vi "Red_Micro_Parse.vi"(10 "Data":string, 11 "Redundant Micro in":T1) -> (3 "Redundant Micro out":T1)   [LabVIEW 2016]
uses:
  type defs/Redundant.ctl
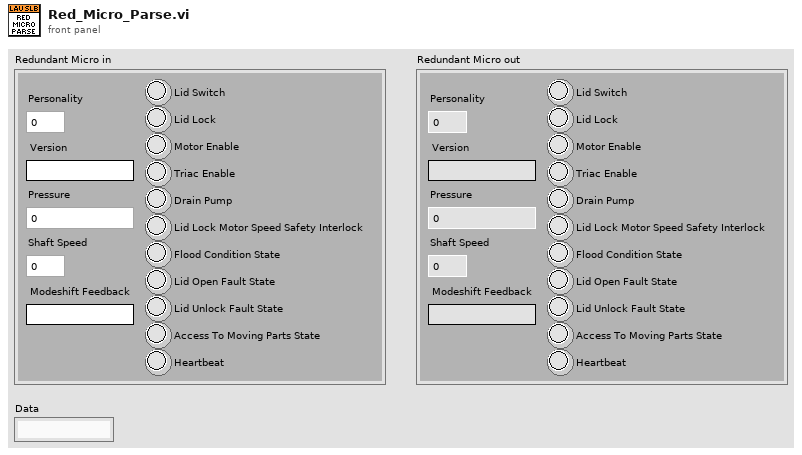
[diagram p1: front panel]
types:
  T1 = typedef "Redundant.ctl" = cluster{"Version":string, "Personality":u8, "Pressure ":dbl, "Shaft Speed":u16, "Modeshift Feedback":string, "Lid Switch":bool, "Lid Lock":bool, "Triac Enable":bool, "Drain Pump":bool, "Lid Lock Motor Speed Safety Interlock":bool, "Flood Condition State":bool, "Lid Open Fault State":bool, "Access To Moving Parts State":bool, "Heartbeat":bool, "Motor Enable":bool, "Lid Unlock Fault State":bool}
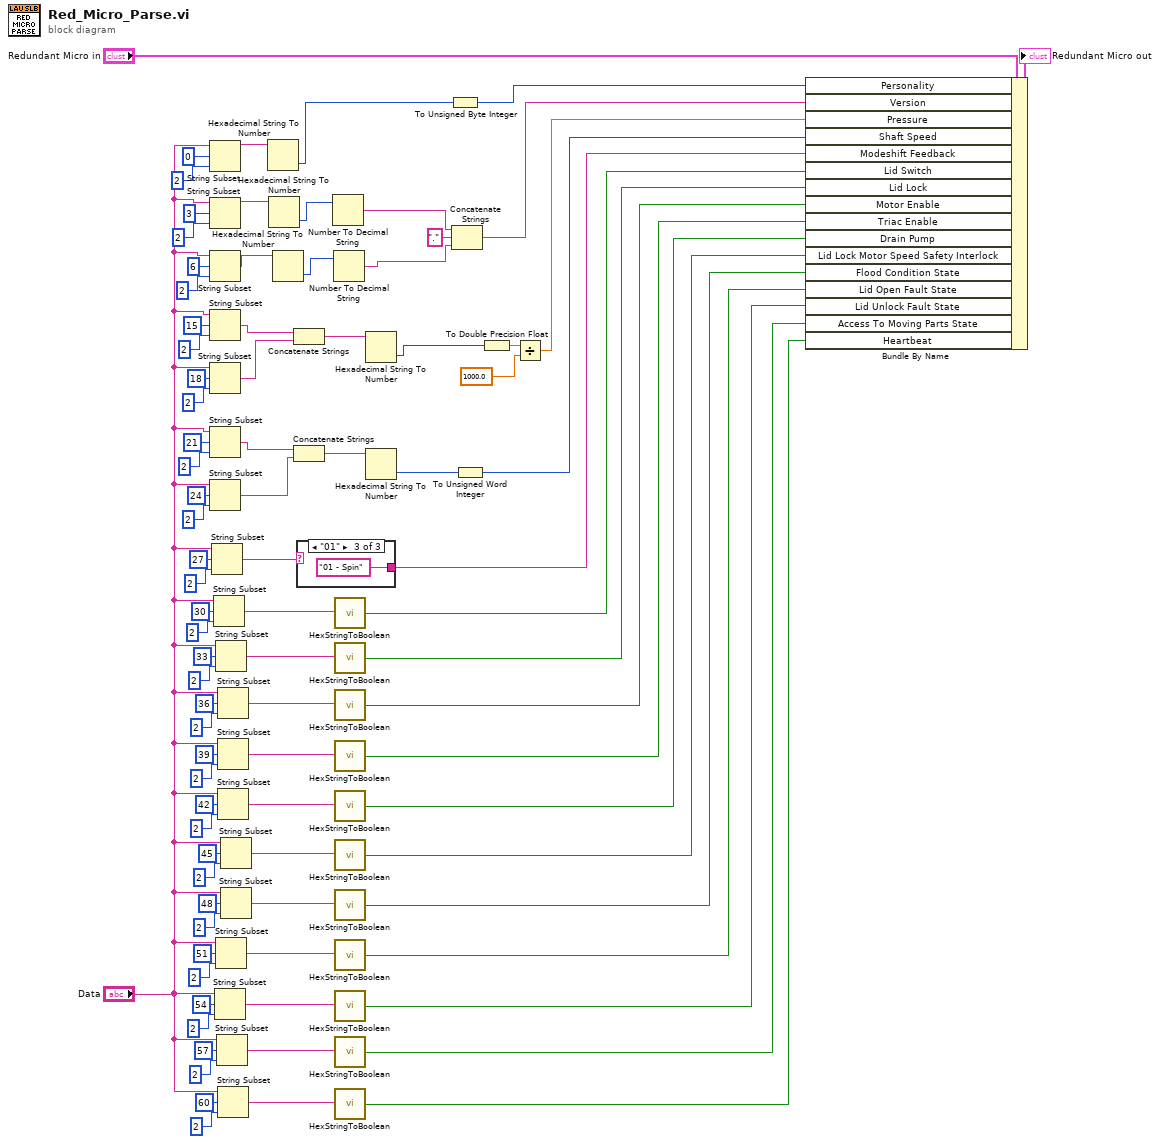
[diagram p0: block diagram]
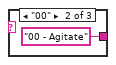
[diagram p3: hidden frame]
diagram:
  n1 = String Subset(string="Data", offset (0)=0, length (rest)=2 ("length (rest)")) -> (substring=w3:string)
  n2 = String Subset(string="Data", offset (0)=3, length (rest)=2 ("length (rest)")) -> (substring=w5:string)
  n3 = String Subset(string="Data", offset (0)=6, length (rest)=2 ("length (rest)")) -> (substring=w11:string)
  n4 = String Subset(string="Data", offset (0)=15, length (rest)=2 ("length (rest)")) -> (substring=w22:string)
  n5 = String Subset(string="Data", offset (0)=18, length (rest)=2 ("length (rest)")) -> (substring=w23:string)
  n6 = String Subset(string="Data", offset (0)=21, length (rest)=2 ("length (rest)")) -> (substring=w31:string)
  n7 = String Subset(string="Data", offset (0)=24, length (rest)=2 ("length (rest)")) -> (substring=w32:string)
  n8 = String Subset(string="Data", offset (0)=27, length (rest)=2 ("length (rest)")) -> (substring=w37:string)
  n9 = String Subset(string="Data", offset (0)=30, length (rest)=2 ("length (rest)")) -> (substring=w41:string)
  n10 = String Subset(string="Data", offset (0)=54, length (rest)=2 ("length (rest)")) -> (substring=w72:string)
  n11 = String Subset(string="Data", offset (0)=33, length (rest)=2 ("length (rest)")) -> (substring=w42:string)
  n12 = String Subset(string="Data", offset (0)=51, length (rest)=2 ("length (rest)")) -> (substring=w60:string)
  n13 = String Subset(string="Data", offset (0)=57, length (rest)=2 ("length (rest)")) -> (substring=w73:string)
  n14 = String Subset(string="Data", offset (0)=36, length (rest)=2 ("length (rest)")) -> (substring=w47:string)
  n15 = String Subset(string="Data", offset (0)=39, length (rest)=2 ("length (rest)")) -> (substring=w48:string)
  n16 = String Subset(string="Data", offset (0)=42, length (rest)=2 ("length (rest)")) -> (substring=w53:string)
  n17 = String Subset(string="Data", offset (0)=60, length (rest)=2 ("length (rest)")) -> (substring=w78:string)
  n18 = String Subset(string="Data", offset (0)=45, length (rest)=2 ("length (rest)")) -> (substring=w54:string)
  n19 = String Subset(string="Data", offset (0)=48, length (rest)=2 ("length (rest)")) -> (substring=w59:string)
  n20 = Hexadecimal String To Number(string=w3) -> (number=w4:u32)  [unwired: 2 in, 1 out]
  n21 = Hexadecimal String To Number(string=w5) -> (number=w12:u32)  [unwired: 2 in, 1 out]
  n22 = Hexadecimal String To Number(string=w11) -> (number=w13:u32)  [unwired: 2 in, 1 out]
  n23 = Concatenate Strings(w22, w23) -> (w24:string)
  n24 = Concatenate Strings(w31, w32) -> (w33:string)
  n25 = case shown="\"01\"" w37 {
    selector: w37 -> [w89 _ _]
    tunnel: [w89 "00 - Agitate" "01 - Spin"] -> w38
    frame Default {
    }
    frame "00" {
    }
    frame "01" {
    }
  }
  n26 = Number To Decimal String(number=w12) -> (decimal integer string=w16:string)  [unwired: 1 in]
  n27 = Number To Decimal String(number=w13) -> (decimal integer string=w15:string)  [unwired: 1 in]
  n28 = call "HexStringToBoolean.vi"("Hex String"=w41) -> ("Boolean"=w63:bool)
  n29 = call "HexStringToBoolean.vi"("Hex String"=w42) -> ("Boolean"=w64:bool)
  n30 = call "HexStringToBoolean.vi"("Hex String"=w47) -> ("Boolean"=w65:bool)
  n31 = call "HexStringToBoolean.vi"("Hex String"=w48) -> ("Boolean"=w66:bool)
  n32 = call "HexStringToBoolean.vi"("Hex String"=w53) -> ("Boolean"=w67:bool)
  n33 = call "HexStringToBoolean.vi"("Hex String"=w54) -> ("Boolean"=w82:bool)
  n34 = call "HexStringToBoolean.vi"("Hex String"=w59) -> ("Boolean"=w68:bool)
  n35 = call "HexStringToBoolean.vi"("Hex String"=w60) -> ("Boolean"=w69:bool)
  n36 = call "HexStringToBoolean.vi"("Hex String"=w72) -> ("Boolean"=w79:bool)
  n37 = call "HexStringToBoolean.vi"("Hex String"=w73) -> ("Boolean"=w80:bool)
  n38 = call "HexStringToBoolean.vi"("Hex String"=w78) -> ("Boolean"=w81:bool)
  n39 = Hexadecimal String To Number(string=w24) -> (number=w25:u32)  [unwired: 2 in, 1 out]
  n40 = Hexadecimal String To Number(string=w33) -> (number=w26:u32)  [unwired: 2 in, 1 out]
  n41 = To Unsigned Byte Integer(number=w4) -> (unsigned 8bit integer=w8:u8)
  n42 = Concatenate Strings(w16, "." ("string"), w15) -> (w17:string)
  n43 = To Unsigned Word Integer(number=w26) -> (unsigned 16bit integer=w34:u16)
  n44 = To Double Precision Float(number=w25) -> (double precision float=w84:dbl)
  n45 = Divide(x=w84, y=1000.0) -> (x/y=w83:dbl)
  n46 = Bundle By Name(cluster="Redundant Micro in", "Personality"=w8, "Version"=w17, "Pressure"=w83, "Shaft Speed"=w34, "Modeshift Feedback"=w38, "Lid Switch"=w63, "Lid Lock"=w64, "Motor Enable"=w65, "Triac Enable"=w66, "Drain Pump"=w67, "Lid Lock Motor Speed Safety Interlock"=w82, "Flood Condition State"=w68, "Lid Open Fault State"=w69, "Lid Unlock Fault State"=w79, "Access To Moving Parts State"=w80, "Heartbeat"=w81) -> (→"Redundant Micro out":T1)
